vi "lab2.2.vi"(8 "y global":dbl[](array[numeric]), 9 "x global":dbl[](array[numeric]) format="%#.6f", 10 "y local":dbl[](array[numeric]), 11 "x local":dbl[](array[numeric])) -> (0 "o":dbl, 1 "a":dbl, 2 "Y0":dbl, 3 "X0":dbl, 4 "resY":dbl[](array[numeric]), 6 "resX":dbl[](array[numeric]))   [LabVIEW 2014]
uses:
  <vilib>/imath/engines/lvmath2/RunTimeEngine/BuiltInFunctions/length/NIMS_length(GV).vi
  <instcachedir>/0/NIMS_length(GV)_08A3D13377FD4E4B96F5795FBF3698FA.lvgen/NIMS_length(GV)_08A3D13377FD4E4B96F5795FBF3698FA_000.vi
  <vilib>/imath/engines/lvmath2/RunTimeEngine/BuiltInFunctions/sum/NIMS_sum(GV).vi
  <instcachedir>/0/NIMS_sum(GV)_67F5EC36BC034E54A6BEC5B0673C00E5.lvgen/NIMS_sum(GV)_67F5EC36BC034E54A6BEC5B0673C00E5_000.vi
  <vilib>/imath/engines/lvmath2/RunTimeEngine/ArithmeticOperatorToken/NIMS_ArithmeticOperator_times.vi
  <instcachedir>/0/NIMS_ArithmeticOperator_times_2EFF5B13FCA4492A81D59089AD809F54.lvgen/NIMS_ArithmeticOperator_times_2EFF5B13FCA4492A81D59089AD809F54_000.vi
  <vilib>/imath/engines/lvmath2/RunTimeEngine/ArithmeticOperatorToken/NIMS_ArithmeticOperator_plus.vi
  <instcachedir>/0/NIMS_ArithmeticOperator_plus_48D6EAACA5D645B09F7EC9C016C2DEA8.lvgen/NIMS_ArithmeticOperator_plus_48D6EAACA5D645B09F7EC9C016C2DEA8_004.vi
  <vilib>/imath/engines/lvmath2/RunTimeEngine/ArithmeticOperatorToken/NIMS_ArithmeticOperator_minus.vi
  <instcachedir>/0/NIMS_ArithmeticOperator_minus_39C0593E74DA4138ACA2AB742906488D.lvgen/NIMS_ArithmeticOperator_minus_39C0593E74DA4138ACA2AB742906488D_003.vi
  <vilib>/imath/engines/lvmath2/RunTimeEngine/ErrorHandling/NIMS_Create Error From Enums.vi
  <vilib>/imathl/engines/lvmath/Functions/Error Handling/Create Error.vi
  <vilib>/imath/engines/lvmath2/RunTimeEngine/NodeEndStatement/NIMS_NodeEndStatement_Output.vi
  <instcachedir>/0/NIMS_NodeEndStatement_Output_53EC0D466D134D7ABD903AC30B43404B.lvgen/NIMS_NodeEndStatement_Output_53EC0D466D134D7ABD903AC30B43404B_010.vi
  <instcachedir>/0/NIMS_NodeEndStatement_Output_53EC0D466D134D7ABD903AC30B43404B.lvgen/NIMS_NodeEndStatement_Output_53EC0D466D134D7ABD903AC30B43404B_005.vi
  <instcachedir>/0/NIMS_NodeEndStatement_Output_53EC0D466D134D7ABD903AC30B43404B.lvgen/NIMS_NodeEndStatement_Output_53EC0D466D134D7ABD903AC30B43404B_001.vi
  <vilib>/imath/engines/lvmath2/RunTimeEngine/ErrorHandling/NIMS_Finalize Error.vi
panel:
  out "m":cdb
  out "Ynew":dbl[](array[numeric])
  out "Xnew":dbl[](array[numeric])
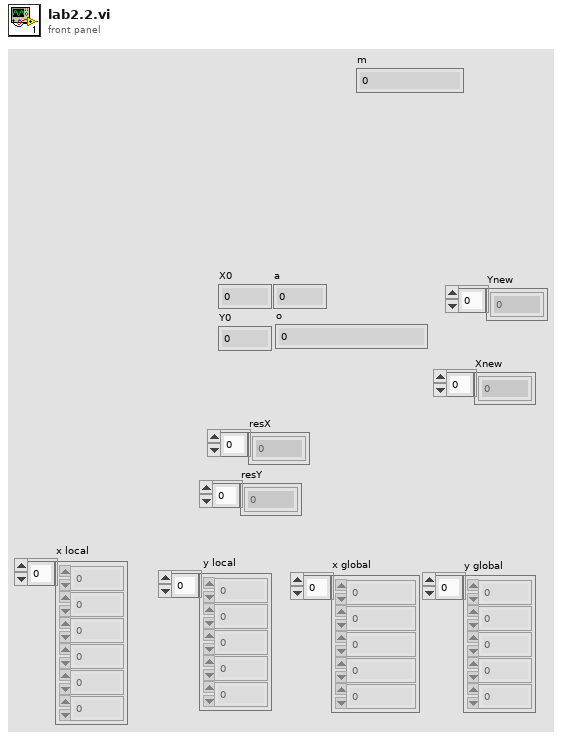
[diagram p1: front panel]
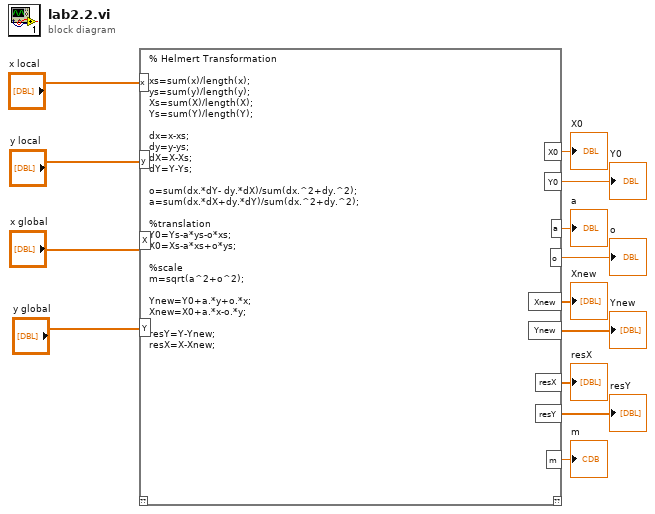
[diagram p0: block diagram]
diagram:
  n1 = mathscript code="% Helmert Transformation\n\nxs=sum(x)/length(x);\nys=sum(y)/length(y);\nXs=sum(X)/length(X);\nYs=sum(Y)/length(Y);\n\ndx=x-xs;\ndy=y-ys;\ndX=X-Xs;\ndY=Y-Ys;\n\no=sum(dx.*dY- dy.*dX)/sum(dx.^2+dy.^2);\na=sum(dx.*dX+dy.*dY)/sum(dx.^2+dy.^2);\n\n%translation\nY0=Ys-a*ys-o*xs;\nX0=Xs-a*xs+o*ys;\n\n%scale\nm=sqrt(a^2+o^2);\n\nYnew=Y0+a.*y+o.*x;\nXnew=X0+a.*x-o.*y;\n\nresY=Y-Ynew;\nresX=X-Xnew;"("x"="x local", "y"="y local", "X"="x global", "Y"="y global") -> ("X0"=→"X0":dbl, "Y0"=→"Y0":dbl, "a"=→"a":dbl, "o"=→"o":dbl, "Xnew"=→"Xnew":dbl[], "Ynew"=→"Ynew":dbl[], "resX"=→"resX":dbl[], "resY"=→"resY":dbl[], "m"=→"m":cdb)  [unwired: 1 in, 1 out]
